vi "TDMS to Patch Image.vi"(0 "Experiment Path":path, 1 "Old Version":bool, 11 "error in (no error)":errorcluster, 12 "Imaging Protocol":T2=enum."Functional Acquisition", 13 "Predominant ROI type":T1=enum."Rectangle", 14 "No of Patches in Experiment":i32) -> (4 "Current Trial Number":i32, 6 "Cancelled":bool, 10 "All Files in Dir":path[](array[path]), 15 "error out":errorcluster)   [LabVIEW 2017]
uses:
  Globals/gl_funct TIFF export globals.vi
  Typedefs/Imaging Protocols enum.ctl
  Typedefs/ROI ID Enum.ctl
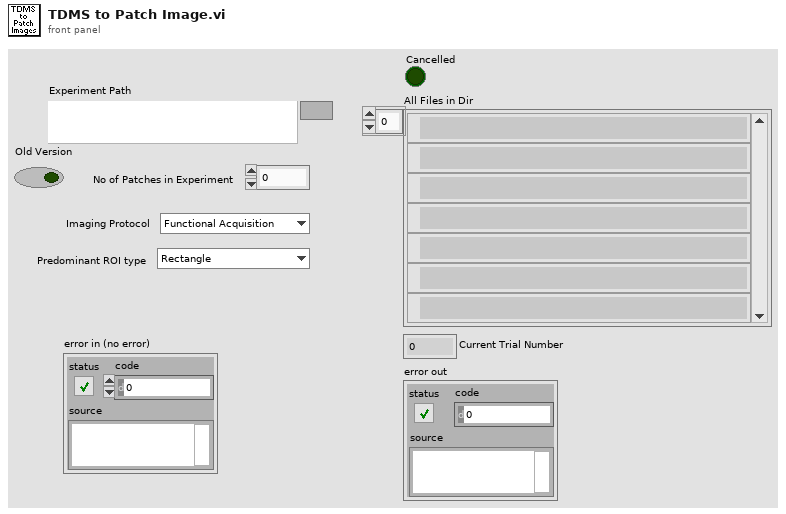
[diagram p1: front panel]
types:
  T1 = typedef "ROI ID Enum.ctl" = enum16{"Point", "MiniScan", "Comp. MiniScan", "Rectangle", "Comp. volume", "Arb. plane point", "None"}
  T2 = typedef "Imaging Protocols enum.ctl" = enum16{"AOL Z-Stack", "Motor Z Stack", "Functional Acquisition", "Single Plane Acquisition", "Volume Acquisition", "Live Imaging", "Live Plane Imaging", "Live Volume Imaging"}
  T3 = typedef "Funct TIFF exporter ctrl refs.ctl" = cluster{"This VI":refnum<vi>, "Current Experiment":refnum<vi>, "Imaging protocol":refnum<vi>, "Predominant ROI type":refnum<vi>, "Patches in Experiment":refnum<vi>, "Folder Path":refnum<vi>, "Export":refnum<vi>, "Trial number":refnum<vi>, "Output TIFF type":refnum<vi>}
  T4 = typedef "Exported TIFF type.ctl" = enum16{"One multi-page TIFF file for each rectangle", "Individual TIFF files"}
  T5 = typedef "Fixed strings.ctl" = cluster{"ROI file name":string, "Normalised ROI file name":string, "Zplane Pockels values file name":string, "Functional data folder name":string, "Experiment Header file name":string, "Z-stack images folder name":string, "Groups setup rel. path":string, "Groups text file rel. path":string, "TDMS files folder name (F.img)":string, "TDMS files folder name (V.acq)":string, "TDMS files folder name (Pl.acq)":string, "Cycle rel times sequence file":string, "Dynamically called VIs folder name":string, "Time Series folder base name":string}
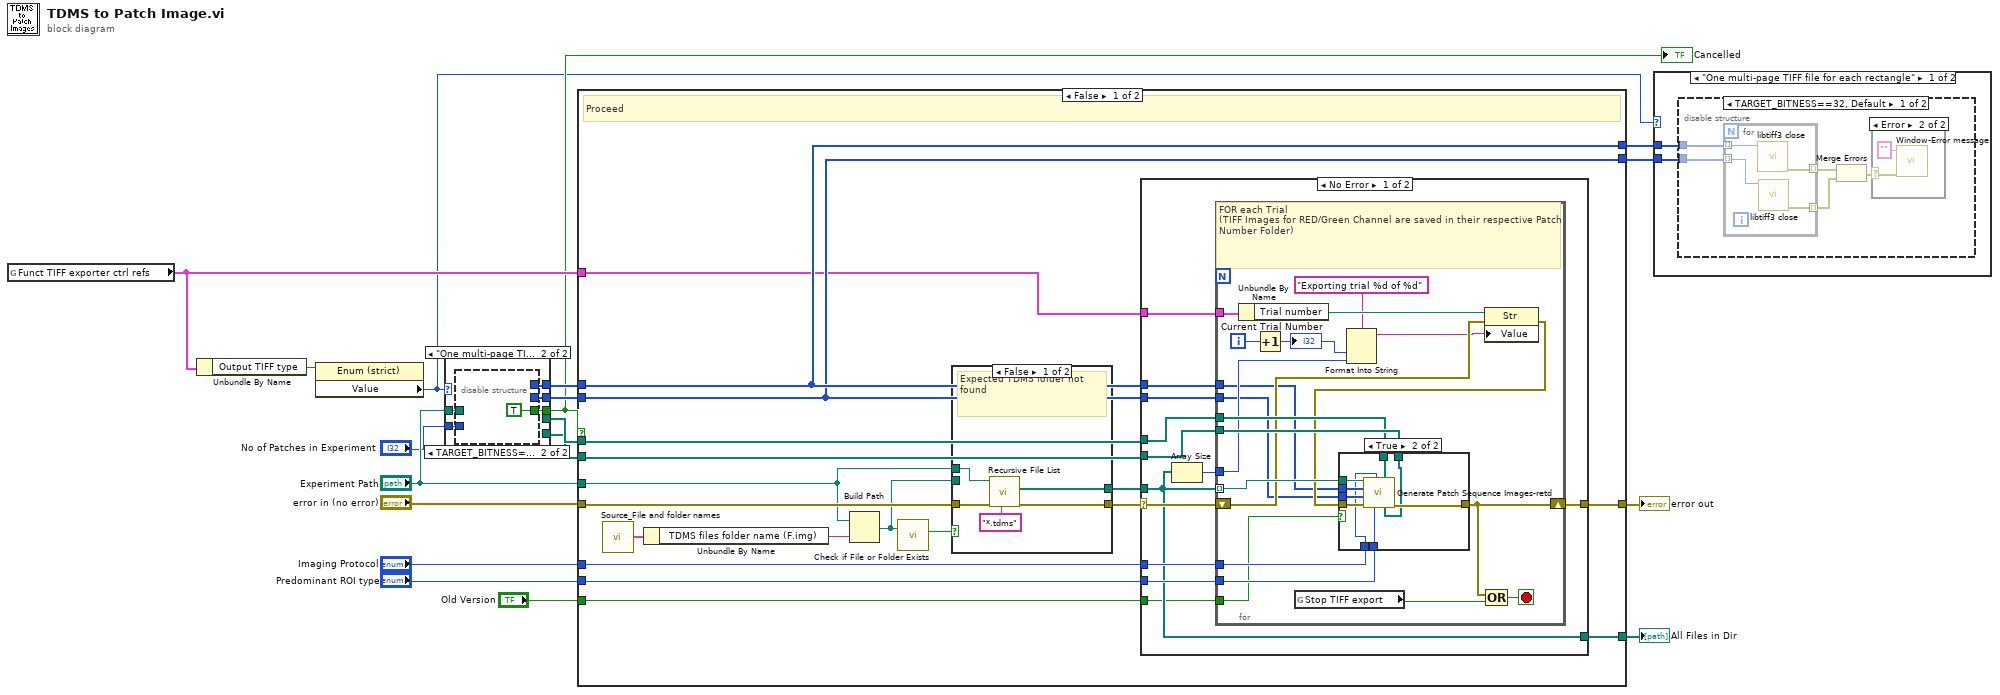
[diagram p0: block diagram]
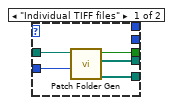
[diagram p5: hidden frame]
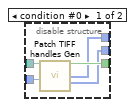
[diagram p6: hidden frame]
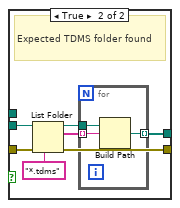
[diagram p7: hidden frame]
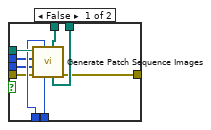
[diagram p8: hidden frame]
diagram:
  n1 = global read "gl_funct TIFF export globals.vi" "Funct TIFF exporter ctrl refs"() -> (w4:T3)
  n2 = Unbundle By Name(w4) -> ("Output TIFF type"=w5:refnum<vi>)
  n3 = property class="Enum (strict)"(reference=w5) -> ("Value"=w2:T4)  [unwired: 1 in, 2 out]
  n4 = case shown="\"One multi-page TIFF file for each rectangle\", Default" w2 {
    tunnel: [w23 _] -> w18
    tunnel: [w22 _] -> w17
    tunnel: [w21 w28] -> w3
    tunnel: "Experiment Path" -> [w20 w27]
    tunnel: "No of Patches in Experiment" -> [w19 w26]
    tunnel: [_ w25] -> w9
    tunnel: [_ w24] -> w8
    frame "Individual TIFF files" {
      n5 = call "Patch Folder Gen.vi"("No of Patches"=w19, "Experimental Folder"=w20) -> ("Green"=w22:path[], "Red"=w23:path[], "Cancelled"=w21:bool)  [unwired: 7 in]
    }
    frame "One multi-page TIFF file for each rectangle", Default {
      n6 = disable-structure shown="TARGET_BITNESS==64" {
        disable-tunnel: [w33 TRUE ("Cancelled")] -> w28
        disable-tunnel: w27 -> [w32 _]
        disable-tunnel: w26 -> [w31 _]
        disable-tunnel: [w30 _] -> w25
        disable-tunnel: [w29 _] -> w24
        frame condition #0 {
          n7 = call "Patch TIFF handles Gen.vi"("Experimental Folder"=w32, "No of Patches"=w31) -> ("Cancelled"=w33:bool, "Red TIFF handles"=w30:i32[], "Green TIFF handles"=w29:i32[])  [unwired: 9 in, 2 out]
        }
        frame condition #1 (active) {
        }
      }
    }
  }
  "Cancelled" <- w3
  n8 = case shown="False" w3 {
    tunnel: w18 -> [w52 _]
    tunnel: w17 -> [w51 _]
    tunnel: "Imaging Protocol" -> [w50 _]
    tunnel: "Predominant ROI type" -> [w49 _]
    tunnel: [w48 w121] -> w13
    tunnel: "error in (no error)" -> [w46 w121]
    tunnel: [w47 _] -> w12
    tunnel: "Experiment Path" -> [w39 _]
    tunnel: w9 -> [w38 w120]
    tunnel: w8 -> [w37 w119]
    tunnel: [w38 w120] -> w7
    tunnel: [w37 w119] -> w6
    tunnel: w4 -> [w36 _]
    tunnel: "Old Version" -> [w35 _]
    frame False {
      # "Proceed"
      n9 = call "Source_File and folder names.vi"() -> ("Fixed strings"=w43:T5)  [unwired: 1 in]
      n10 = Unbundle By Name(w43) -> ("TDMS files folder name (F.img)"=w42:string)
      n11 = Build Path(base path=w39, name or relative path=w42) -> (appended path=w40:path)
      n12 = call <vilib>:"Check if File or Folder Exists.vi"("path"=w40) -> ("file or folder exists?"=w41:bool)  [unwired: 8 in, 2 out]
      n13 = case shown="False" w41 {
        tunnel: w46 -> [w57 w64]
        tunnel: [w56 w63] -> w45
        tunnel: [w55 w58] -> w44
        tunnel: w40 -> [_ w62]
        tunnel: w39 -> [w53 _]
        frame False {
          # "Expected TDMS folder not found"
          n14 = call <vilib>:"Recursive File List.vi"("pattern"="*.tdms", "error in (no error)"=w57, "Folder Path"=w53) -> ("error out"=w56:errorcluster, "All Files in Dir"=w55:path[])  [unwired: 4 in, 3 out]
        }
        frame True {
          # "Expected TDMS folder found"
          n15 = List Folder(path=w62, pattern="*.tdms", error in=w64) -> (path out=w59:path, filenames=w60:string[], error out=w63:errorcluster)  [unwired: 1 in, 1 out]
          n16 = for {
            tunnel: w60 -> [w66] mode=indexing
            tunnel: w59 -> [w67]
            tunnel: [w65] -> w58 mode=indexing
            n17 = Build Path(base path=w67, name or relative path=w66) -> (appended path=w65:path)
          }
        }
      }
      n18 = case shown="No Error" w45 {
        selector: w45 -> [w74 w118]
        tunnel: w44 -> [w72 _]
        tunnel: w52 -> [w79 _]
        tunnel: w51 -> [w78 _]
        tunnel: w50 -> [w77 _]
        tunnel: w49 -> [w76 _]
        tunnel: [w75 w118] -> w48
        tunnel: [w72 _] -> w47
        tunnel: w36 -> [w73 _]
        tunnel: w38 -> [w70 _]
        tunnel: w37 -> [w69 _]
        tunnel: w35 -> [w68 _]
        frame No Error {
          n19 = Array Size(array=w72) -> (size(s)=w71:i32)
          n20 = for {
            tunnel: w72 -> [w99] mode=indexing
            tunnel: w79 -> [w97]
            tunnel: w78 -> [w98]
            tunnel: w77 -> [w96]
            tunnel: w76 -> [w95]
            shift-right: [w92] -> w75
            shift-left: w74 -> [w89]
            tunnel: w73 -> [w91]
            tunnel: w71 -> [w85]
            tunnel: w70 -> [w83]
            tunnel: w69 -> [w82]
            tunnel: w68 -> [w80]
            i -> [w81]
            stop <- w93 stop-if-true
            # "FOR each Trial\n(TIFF Images for RED/Green Channel are saved in their respective Patch Number Folder)"
            n21 = Unbundle By Name(w91) -> ("Trial number"=w90:refnum<vi>)
            n22 = Increment(x=w81) -> (x+1=w86:i32)
            "Current Trial Number" <- w86
            n23 = global read "gl_funct TIFF export globals.vi" "Stop TIFF export"() -> (w94:bool)
            n24 = Format Into String(format string="Exporting trial %d of %d", w86, w85) -> (resulting string=w84:string)  [unwired: 2 in, 1 out]
            n25 = property class="Str"(reference=w90, error in=w89, "Value"=w84) -> (error out=w88:errorcluster)  [unwired: 1 out]
            n26 = case shown="True" w80 {
              tunnel: w99 -> [w108 w113]
              tunnel: w98 -> [w107 w114]
              tunnel: w97 -> [w106 w115]
              tunnel: w96 -> [w105 w110]
              tunnel: w95 -> [w104 w109]
              tunnel: [w103 w116] -> w92
              tunnel: w88 -> [w102 w117]
              tunnel: w83 -> [w101 w112]
              tunnel: w82 -> [w100 w111]
              frame False {
                n27 = call "Generate Patch Sequence Images.vi"("Green"=w107, "Red"=w106, "Predominant ROI type"=w104, "Imaging Protocol"=w105, "error in (no error)"=w102, "Green TIFF handles"=w100, "Red TIFF handles"=w101, "TDMS file path & name"=w108) -> ("error out"=w103:errorcluster)  [unwired: 2 in, 1 out]
              }
              frame True {
                n28 = call "Generate Patch Sequence Images-retd.vi"("Green"=w114, "Red"=w115, "Predominant ROI type"=w109, "Imaging Protocol"=w110, "error in (no error)"=w117, "Green TIFF handles"=w111, "Red TIFF handles"=w112, "TDMS file path & name"=w113) -> ("error out"=w116:errorcluster)  [unwired: 2 in, 1 out]
              }
            }
            n29 = Compound Arithmetic op=OR(w92, w94) -> (w93:bool)
          }
        }
        frame Error {
        }
      }
    }
    frame True {
      # "Error or cancelled"
    }
  }
  "error out" <- w13
  "All Files in Dir" <- w12
  n30 = case shown="\"One multi-page TIFF file for each rectangle\"" w2 {
    tunnel: w7 -> [w123 _]
    tunnel: w6 -> [w122 _]
    frame "One multi-page TIFF file for each rectangle" {
      n31 = disable-structure shown="TARGET_BITNESS==32, Default" {
        disable-tunnel: w123 -> [w128 _]
        disable-tunnel: w122 -> [w127 _]
        frame condition #0 {
          n32 = for {
            tunnel: w128 -> [w134] mode=indexing
            tunnel: w127 -> [w133] mode=indexing
            tunnel: [w132] -> w125 mode=indexing
            tunnel: [w131] -> w126 mode=indexing
            n33 = call "libtiff3 close.vi"("Handle"=w134) -> ("error out"=w131:errorcluster)  [unwired: 9 in]
            n34 = call "libtiff3 close.vi"("Handle"=w133) -> ("error out"=w132:errorcluster)  [unwired: 9 in]
          }
          n35 = Merge Errors(w126, w125) -> (w124:errorcluster)
          n36 = case shown="Error" w124 {
            selector: w124 -> [_ w130]
            frame No Error {
            }
            frame Error {
              n37 = call "Window-Error message.vi"("error in (no error)"=w130, "Message"="") -> ()  [unwired: 9 in, 1 out]
            }
          }
        }
        frame condition #1 (active) {
        }
      }
    }
    frame "Individual TIFF files", Default {
    }
  }
